vi "Voc_libary.vi"(10 "Current":sgl[](array[numeric]), 11 "Voltage":sgl[](array[numeric])) -> (3 "Voc":sgl)   [LabVIEW 2013]
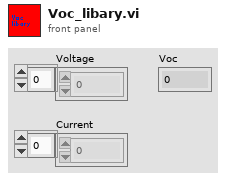
[diagram p1: front panel]
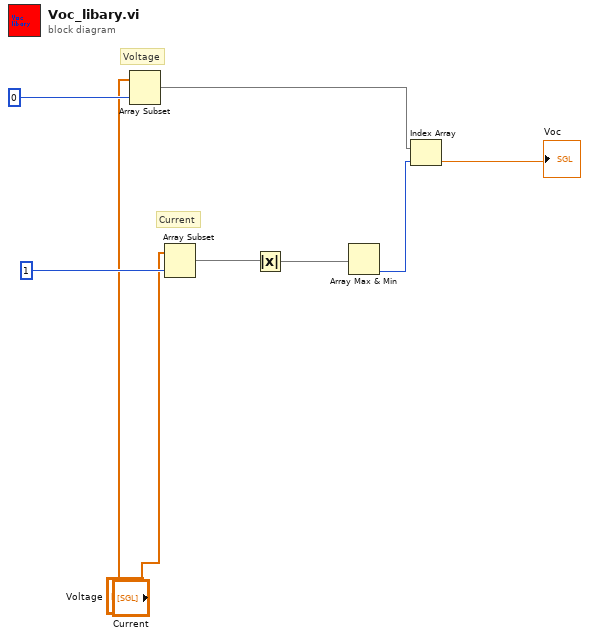
[diagram p0: block diagram]
diagram:
  # "Current"
  # "Voltage"
  n1 = Array Subset(array="Voltage", length=0 ("index")) -> (w7:sgl[])  [unwired: 1 in]
  n2 = Array Subset(array="Current", length=1 ("index")) -> (w5:sgl[])  [unwired: 1 in]
  n3 = Absolute Value(x=w5) -> (abs(x)=w6:sgl[])
  n4 = Array Max & Min(array=w6) -> (min index (indices)=w8:i32)  [unwired: 3 out]
  n5 = Index Array(array=w7, index=w8) -> (element=→"Voc":sgl)
